vi "ex7-1.vi"   [LabVIEW 2013]
uses:
  <vilib>/NXT/Block Support/NXT_InputPort.ctl
  <vilib>/NXT/Dual Mode Library/Sensors/Touch_Bumped.vi
  <vilib>/NXT/Dual Mode Library/Display/drawNumber.vi
types:
  T1 = typedef "NXT_InputPort.ctl" = u32
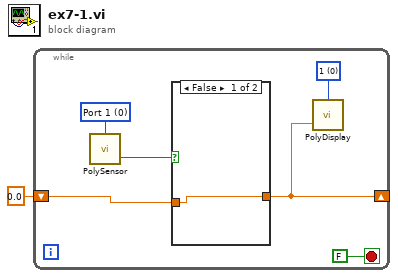
[diagram p0: block diagram]
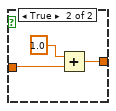
[diagram p2: hidden frame]
diagram:
  n1 = while {
    shift-right: [w3] -> _
    shift-left: 0.0 -> [w5]
    stop <- FALSE stop-if-true
    w4 = i16 0 items=["1", "2", "3", "4", "5", "6", "7", "8", "9", "10", "11", "12"] ("Line")
    w6 = T1 0 items=["Port 1", "Port 2", "Port 3", "Port 4"] ("Port (Port 1)")
    n2 = call-poly <vilib>:"PolySensor.vi"("Port (Port 1)"=w6) -> ("Yes / No"=w7:bool)  [unwired: 2 in, 1 out]
    n3 = case shown="False" w7 {
      tunnel: w5 -> [w8 w10]
      tunnel: [w8 w9] -> w3
      frame False {
      }
      frame True {
        n4 = Add(x=1.0, y=w10) -> (x+y=w9:dbl)
      }
    }
    n5 = call-poly <vilib>:"PolyDisplay.vi"("number"=w3, "Line"=w4) -> ()  [unwired: 2 in, 1 out]
  }
